vi "GetAcquisitionData.vi"(8 "error in":errorcluster, 9 "To":i32, 10 "From":i32, 11 "connection ID in":refnum<k5>) -> (0 "error out":errorcluster, 1 "Error Info":T1, 2 "Data":dbl[](array[numeric]), 3 "connection ID out":refnum<k5>, 4 "Log String":string)   [LabVIEW 2020, in "ProdigyRemoteControl.lvlib"]
uses:
  ProdigyRemoteControl.lvlib
  DEFINITIONS/DEF_RcError.ctl
  DEFINITIONS/DEF_RcCmd.ctl
panel:
  out "OK":bool
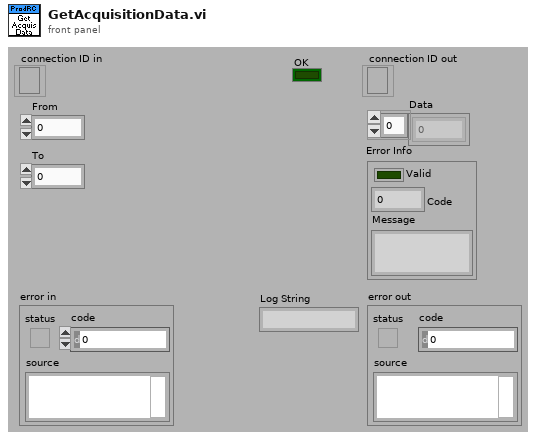
[diagram p1: front panel]
types:
  T1 = typedef "ProdigyRemoteControl.lvlib/DEF_RcError.ctl" = cluster{"Valid":bool, "Code":u16, "Message":string}
  T2 = typedef "ProdigyRemoteControl.lvlib/DEF_RcCmd.ctl" = string
  T3 = enum16{"Standard", "Buffered", "CRLF", "Immediate"}
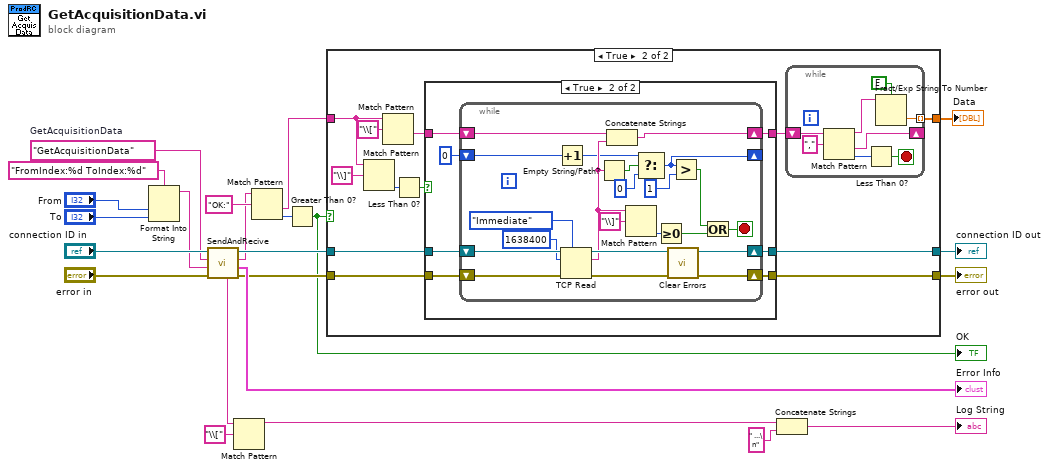
[diagram p0: block diagram]
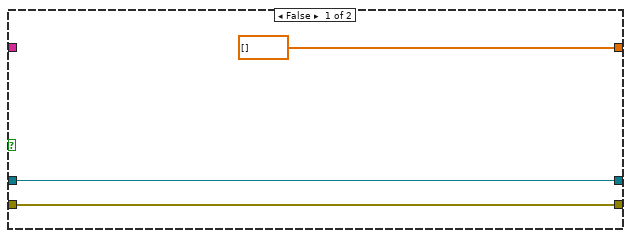
[diagram p2: hidden frame]
diagram:
  w21 = T2 "GetAcquisitionData"  # GetAcquisitionData
  n1 = Format Into String(format string="FromIndex:%d ToIndex:%d", "From", "To") -> (resulting string=w20:string)  [unwired: 2 in, 1 out]
  n2 = call "SendAndRecive.vi"("error in"="error in", "Parameters"=w20, "Command"=w21, "connection ID in"="connection ID in") -> ("error out"=w6:errorcluster, "Error Info"=→"Error Info":T1, "Answer"=w3:string, "connection ID out"=w7:refnum<k5>, "Log String"=w13:string)  [unwired: 3 in]
  n3 = Match Pattern(string=w13, regular expression="\\[") -> (before substring=w12:string)  [unwired: 1 in, 3 out]
  n4 = Match Pattern(string=w3, regular expression="OK:") -> (after substring=w2:string, offset past match=w8:i32)  [unwired: 1 in, 2 out]
  n5 = Greater Than 0?(x=w8) -> (x > 0?=w1:bool)
  "OK" <- w1
  n6 = case shown="True" w1 {
    tunnel: [dbl[] [] w38] -> w15
    tunnel: w7 -> [w26 w37]
    tunnel: w6 -> [w25 w36]
    tunnel: [w26 w35] -> w5
    tunnel: [w25 w34] -> w4
    tunnel: w2 -> [_ w29]
    frame False {
    }
    frame True {
      n7 = Match Pattern(string=w29, regular expression="\\]") -> (offset past match=w30:i32)  [unwired: 1 in, 3 out]
      n8 = Match Pattern(string=w29, regular expression="\\[") -> (after substring=w32:string)  [unwired: 1 in, 3 out]
      n9 = Less Than 0?(x=w30) -> (x < 0?=w28:bool)
      n10 = case shown="True" w28 {
        tunnel: w37 -> [w40 w48]
        tunnel: w36 -> [w39 w47]
        tunnel: [w40 w46] -> w35
        tunnel: [w39 w44] -> w34
        tunnel: w32 -> [w41 w43]
        tunnel: [w41 w42] -> w27
        frame False {
        }
        frame True {
          n11 = while {
            shift-right: [w65] -> w46
            shift-left: w48 -> [w69]
            shift-right: [w49] -> w44
            shift-left: w47 -> [w68]
            shift-right: [w63] -> w42
            shift-left: w43 -> [w64]
            shift-right: [w53] -> _
            shift-left: 0 -> [w55]
            stop <- w58 stop-if-true
            n12 = Increment(x=w55) -> (x+1=w56:i32)
            n13 = TCP Read(connection ID=w69, bytes to read=1638400, error in (no error)=w68, 7:T3."Immediate" ("mode (standard)")) -> (connection ID out=w65:refnum<k5>, data out=w61:string, error out=w50:errorcluster)  [unwired: 1 in]
            n14 = Empty String/Path?(string/path=w61) -> (empty?=w57:bool)
            n15 = Concatenate Strings(w64, w61) -> (w63:string)
            n16 = Match Pattern(string=w61, regular expression="\\]") -> (offset past match=w60:i32)  [unwired: 1 in, 3 out]
            n17 = Select(t=w56, s=w57, f=0) -> (s? t:f=w53:i32)
            n18 = Greater Or Equal To 0?(x=w60) -> (x >= 0?=w59:bool)
            n19 = call <vilib>:"Clear Errors.vi"("error in (no error)"=w50) -> ("error out"=w49:errorcluster)  [unwired: 5 in, 1 out]
            n20 = Greater?(x=w53, y=1) -> (0:w52:bool)
            n21 = Or(x=w52, y=w59) -> (x .or. y?=w58:bool)
          }
        }
      }
      n22 = while {
        shift-right: [w75] -> _
        shift-left: w27 -> [w77]
        tunnel: [w72] -> w38 mode=indexing
        stop <- w73 stop-if-true
        n23 = Match Pattern(string=w77, regular expression=",") -> (before substring=w71:string, after substring=w75:string, offset past match=w74:i32)  [unwired: 1 in, 1 out]
        n24 = Less Than 0?(x=w74) -> (x < 0?=w73:bool)
        n25 = Fract/Exp String To Number(use system decimal point (T)=FALSE, string=w71) -> (number=w72:dbl)  [unwired: 2 in, 1 out]
      }
    }
  }
  "connection ID out" <- w5
  "error out" <- w4
  "Data" <- w15
  n26 = Concatenate Strings(w12, " ...\n" ("string")) -> (→"Log String":string)
